vi "new.vi"() -> ()   [LabVIEW 2012, in "StimulCtrls.lvlib"]
uses:
  StimulCtrls.lvlib
  Program.lvclass
panel:
  in  "PRG out":refnum<class "Program.lvclass">
  in  "PRG in":refnum<class "Program.lvclass">
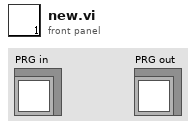
[diagram p1: front panel]
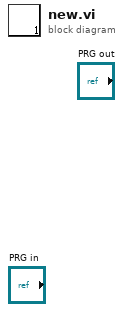
[diagram p0: block diagram]
diagram:
